vi "Read Connections.vi"(8 "error in (no error)":errorcluster, 11 "PID in":refnum<class "INL PID.lvclass">) -> (0 "error out":errorcluster, 2 "Integrator DAQ Channels":T1={"V0"="cDAQ1Mod1/ai0", "S1"="cDAQ1Mod5/port0/line4", "S2"="cDAQ1Mod5/ctr0"}, 3 "PID out":refnum<class "INL PID.lvclass">)   [LabVIEW 2011, in "INL PID.lvclass"]
uses:
  INL PID.lvclass
  Integrator DAQmx Channels.ctl
  INL PID.lvclass/INL PID.ctl
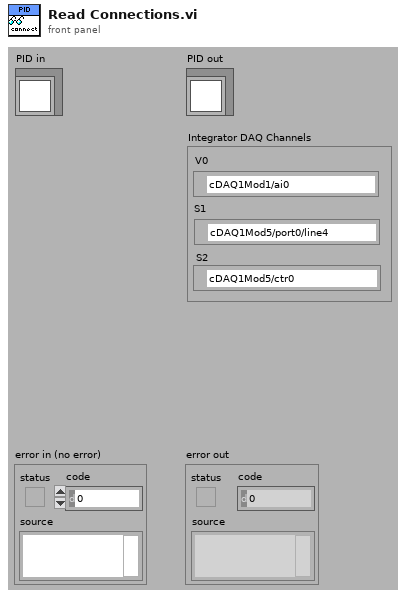
[diagram p1: front panel]
types:
  T1 = typedef "INL PID.lvclass/Integrator DAQmx Channels.ctl" = cluster{"V0":tag, "S1":tag, "S2":tag}
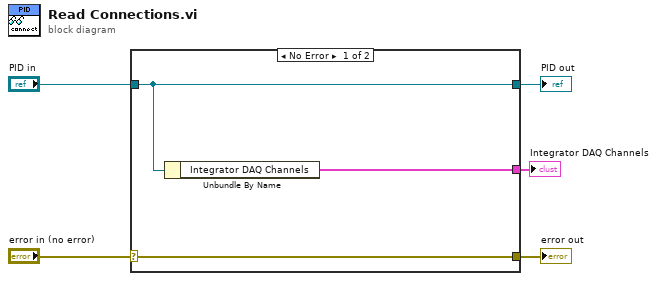
[diagram p0: block diagram]
diagram:
  n1 = case shown="No Error" "error in (no error)" {
    selector: "error in (no error)" -> [w8 w9]
    tunnel: [w8 w9] -> w4
    tunnel: [w7 w10] -> w2
    tunnel: "PID in" -> [w7 w10]
    tunnel: [w6 _] -> w1
    frame No Error {
      n2 = Unbundle By Name(w7) -> ("Integrator DAQ Channels"=w6:T1)
    }
    frame Error {
    }
  }
  "error out" <- w4
  "PID out" <- w2
  "Integrator DAQ Channels" <- w1
